vi "Requests.vi"(8 "error in (no error)":errorcluster, 9 "write enable":bool=TRUE, 11 "SHD in":refnum<class "SHINI SHD.lvclass">) -> (0 "error out":errorcluster, 3 "SHD out":refnum<class "SHINI SHD.lvclass">)   [LabVIEW 2021, in "SHINI SHD.lvclass"]
uses:
  SHINI SHD.lvclass
  D:/my_projects/projects/21/Master CR/Master CR.lvclass
  D:/my_projects/projects/21/Master CR/Devices/ET7000/TCP/TCP.lvclass
  Master CR.lvclass/Master CR.ctl
  Modbus_v121c/Modbus Data Unit/Modbus Data Unit.lvclass/Modbus Data Unit.ctl
  Modbus_v121c/Network Protocol/Network Master/Network Master.lvclass/Network Master.ctl
  Network Protocol/Read Network Protocol.vi
  Modbus_v121c/Master Function Definition/Read Holding Registers Request.vi
  Modbus_v121c/Master Function Definition/Read Holding Registers Response.vi
  Modbus_v121c/Network Protocol/Network Master/Read write Master.vi
  Modbus_v121c/Modbus Data Unit/Construct PDU.vi
  Modbus_v121c/Utility/Bytes to U16s.vi
  Modbus_v121c/Master Function Definition/Function code mismatch error.vi
  Modbus_v121c/Data Model/Error Generator.vi
  Modbus_v121c/Modbus Data Unit/Deconstruct PDU.vi
  ET7000/TCP/TCP.lvclass
  Modbus_v121c/Network Protocol/Network Master/Network Master.lvclass
  Modbus_v121c/Modbus Data Unit/Modbus Data Unit.lvclass
  Modbus_v121c/Data Model/Device Data Model.lvclass
  Modbus_v121c/Transmission Data Unit/Transmission Data Unit.lvclass
  Master CR.lvclass
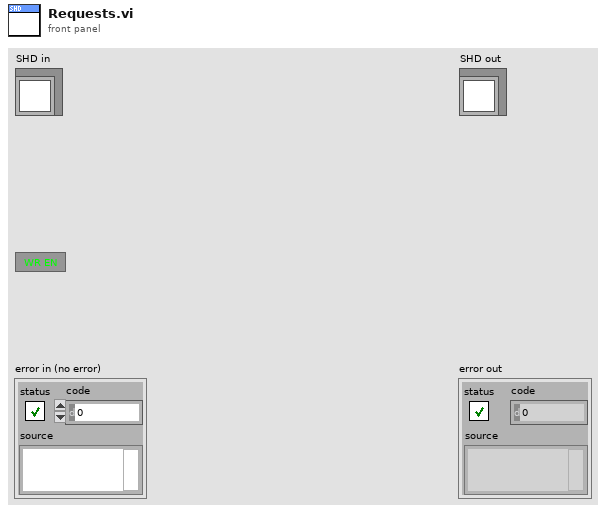
[diagram p1: front panel]
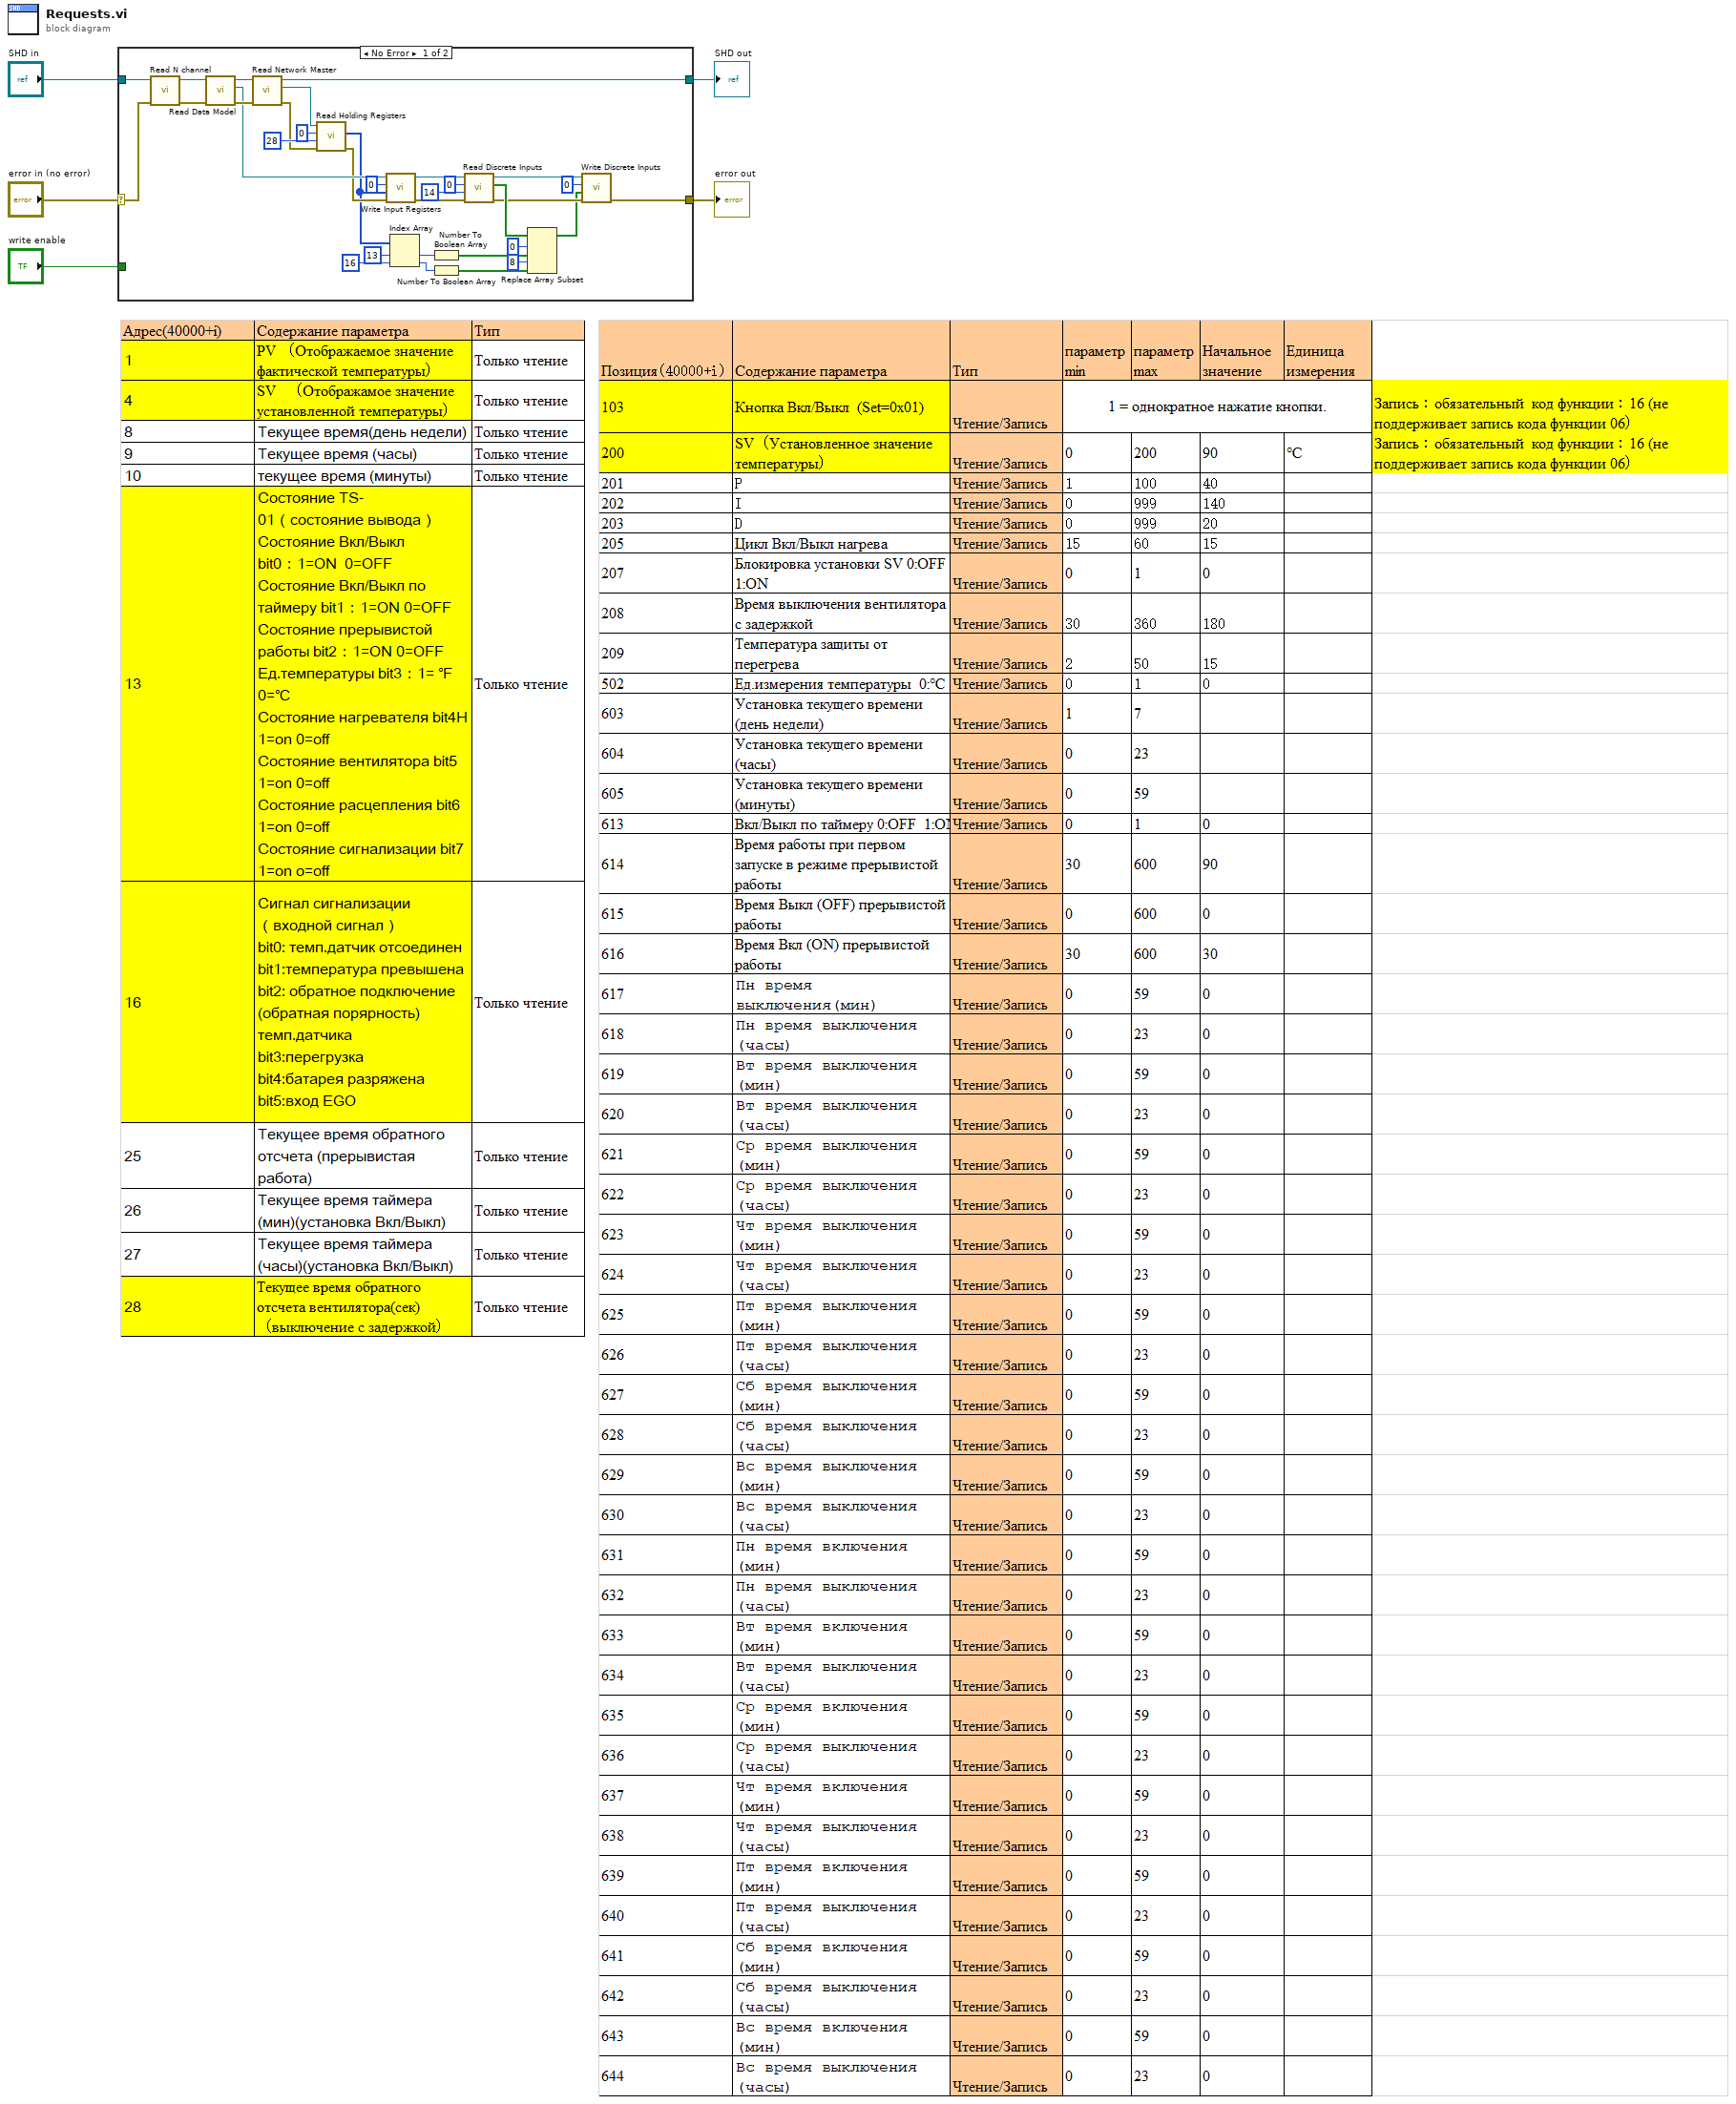
[diagram p0: block diagram]
diagram:
  n1 = case shown="No Error" "error in (no error)" {
    selector: "error in (no error)" -> [w36 w40]
    tunnel: [w7 w40] -> w1
    tunnel: [w6 w39] -> w2
    tunnel: "SHD in" -> [w38 w39]
    tunnel: "write enable" -> [_ _]
    frame No Error {
      n2 = call "Read N channel.vi"("error in (no error)"=w36, "Master CR in"=w38) -> ("error out"=w35:errorcluster, "Master CR out"=w37:refnum<class "SHINI SHD.lvclass">)  [unwired: 7 in, 1 out]
      n3 = call "Read Data Model.vi"("error in (no error)"=w35, "Master CR in"=w37) -> ("error out"=w33:errorcluster, "Data Model"=w27:refnum<class "Device Data Model.lvclass">, "Master CR out"=w34:refnum<class "SHINI SHD.lvclass">)  [unwired: 7 in]
      n4 = call "Read Network Master.vi"("error in (no error)"=w33, "TCP in"=w34) -> ("error out"=w29:errorcluster, "Network Master"=w31:refnum<class "Network Master.lvclass">, "TCP out"=w6:refnum<class "SHINI SHD.lvclass">)  [unwired: 7 in]
      n5 = call "Read Holding Registers.vi"("error in (no error)"=w29, "number of holding registers"=u16 28, "starting address"=u16 0, "Modbus master in"=w31) -> ("error out"=w26:errorcluster, "register values"=w23:u16[])  [unwired: 5 in, 1 out]
      n6 = call-dynamic "Write Input Registers.vi"("error in (no error)"=w26, "register values"=w23, "starting address"=u16 0, "Device Data Model in"=w27) -> ("error out"=w24:errorcluster, "Device Data Model out"=w25:refnum<class "Device Data Model.lvclass">)  [unwired: 6 in]
      n7 = Index Array(array=w23, index #1=13 ("index"), index #2=16 ("index")) -> (element #1=w20:u16, element #2=w19:u16)
      n8 = Number To Boolean Array(number=w20) -> (Boolean array=w14:bool[])
      n9 = Number To Boolean Array(number=w19) -> (Boolean array=w12:bool[])
      n10 = call-dynamic "Read Discrete Inputs.vi"("error in"=w24, "number of inputs"=u16 14, "starting address"=u16 0, "device data model in"=w25) -> ("error out"=w10:errorcluster, "data"=w16:bool[], "device data model out"=w11:refnum<class "Device Data Model.lvclass">)  [unwired: 5 in]
      n11 = Replace Array Subset(array=w16, new element #1=w14, index #1=0 ("index"), new element #2=w12, index #2=8 ("index")) -> (w8:bool[])
      n12 = call-dynamic "Write Discrete Inputs.vi"("error in (no error)"=w10, "input values"=w8, "starting address"=u16 0, "Device Data Model in"=w11) -> ("error out"=w7:errorcluster)  [unwired: 6 in, 1 out]
    }
    frame Error {
    }
  }
  "error out" <- w1
  "SHD out" <- w2
